vi "10-Tap 8-Bit Camera with DRAM(Host).vi"() -> ()   [LabVIEW 2014]
doc: "This is the host VI for the 10-Tap 8-Bit Camera with DRAM example. This example demonstrates how to acquire images from a 10-tap, 8-bit, extended configuration, Camera Link camera and display the images on the host. This example supports area scan and line scan cameras for both continuous and finite acquisitions.\n\nThis example also demonstrates the use of DRAM as a frame buffer for very high speed acquisitions. Data packing and flow-control are also employed to maximize use of the available DRAM and FIFOs in terms of both memory space and performance.\n\nAdditionally, the example demonstrates the serial server, which allows third-party camera configuration utilities to communicate with the camera using the Camera Link serial interface while this VI is running."
uses:
  <vilib>/userdefined/High Color/nirio_resource_hc.ctl
  <vilib>/FPGAPlugInAG/PCIe-1473R/niLvFpga_Open_PCIe-1473R.vi
  <vilib>/rvi/interface/common/dynamic/niFpgaDynamicAddResources.vi
  <vilib>/FPGAPlugInAG/Dynamic/niLvFpga_Reset_Dynamic.vi
  <vilib>/Utility/error.llb/Error Cluster From Error Code.vi
  <vilib>/rvi/errors/niLvFpgaAdjustHostInterfaceError.vi
  <vilib>/FPGAPlugInAG/Dynamic/niLvFpga_Run_Dynamic.vi
  <vilib>/rvi/interface/common/niFpgaWaitOnOcc.vi
  <vilib>/DAQmx/write.llb/DAQmx Write (Analog DBL 1Chan 1Samp).vi
  <vilib>/FPGAPlugInAG/Dynamic/niLvFpga_Close_Dynamic.vi
  <vilib>/rvi/interface/nirviOpenFPGA/nirviOpenFPGA.xnode
  FPGA Bitfiles/10-Tap8-bitCamer_FPGATarget_10-Tap8-bitCamer_C490DC32.lvbitx
  10-Tap 8-Bit Camera with DRAM(FPGA).vi
  <vilib>/rvi/interface/nirviMethod/nirviMethod.xnode
  <vilib>/rvi/interface/nirviReadWriteControl/nirviReadWriteControl.xnode
  <vilib>/rvi/interface/nirviCloseFPGA/nirviCloseFPGA.xnode
  <vilib>/rvi/interface/Simulation/niFpgaSimulationCallBeginRW.vi
  <vilib>/rvi/errors/niLvFpgaMergeErrorWithErrorCode.vi
  NiFpgaLv.dll
  <vilib>/FPGAPlugInAG/Dynamic/niLvFpga_ReadFifo_Dynamic.vi
  <vilib>/FPGAPlugInAG/Dynamic/niLvFpga_ConfigureFifo_Dynamic.vi
  <vilib>/FPGAPlugInAG/Dynamic/niLvFpga_StartFifo_Dynamic.vi
panel:
  out "测得角度":dbl
  out "?":dbl
  out "目标中心":dbl
  out "?":dbl
  out "边框中心":dbl
  in  "BodyLength":dbl=10.0
  in  "FishLength":u16=300
  out "?":u16
  out "?":u16
  out "Xmax":u16
  out "边框":u16
  in  "Y":dbl=384.0 format="%#_13g"
  in  "X":dbl=520.0 format="%#_13g"
  in  "offset":dbl=150.0
  in  "SpeedFactor":dbl=1.0
  out "数量":i32
  out "?":fxp<+,32,16> format="%.21g"
  out "测得中心":fxp<+,32,16> format="%.21g"
  in  "Threshold":u8=96
  in  "DMA Buffer Size\n(In Images)":u32=64 caption="DMA Buffer Size"
  in  "Signal Mapping":T1(ring)=enum."Basler 10-tap"
  out "Acq In Progress":bool
  in  "Line Scan":bool
  in  "Frames To Acquire":u32 caption="Frames To Acquire\n(0 = infinite)"
  in  "Cancel":bool
  out "Acq'd Frame Width":u32
  in  "Stopped":bool
  in  "RIO Device":T2="Horizontal"
  out "DMA Write Timeout":bool
  in  "Start Serial Server":bool=TRUE
  out "Frames Acq'd":u32
  out "Acq'd Frame Height":u32
  out "Image":T3(plugin-control)
  in  "Acquire":bool
  in  "Stop":bool
  in  "Image Height":u32=768 max=65535
  in  "Image Width":u32=1040 max=65535 step=40
  out "Initialized":bool
  # "这个值越小，那么即便是比较小的距离也会移动较快，参考值50"
  # "与速度有关的乘方因子，必须是奇数，参考值1"
  # "目标位置"
  # "期望中心位置"
  # "鱼的身体长度，如果边界大小超过这个值，就放弃此次补偿计算，参考值800"
  # "希望补偿的长度，一般应小于鱼的身体长度，参考值10"
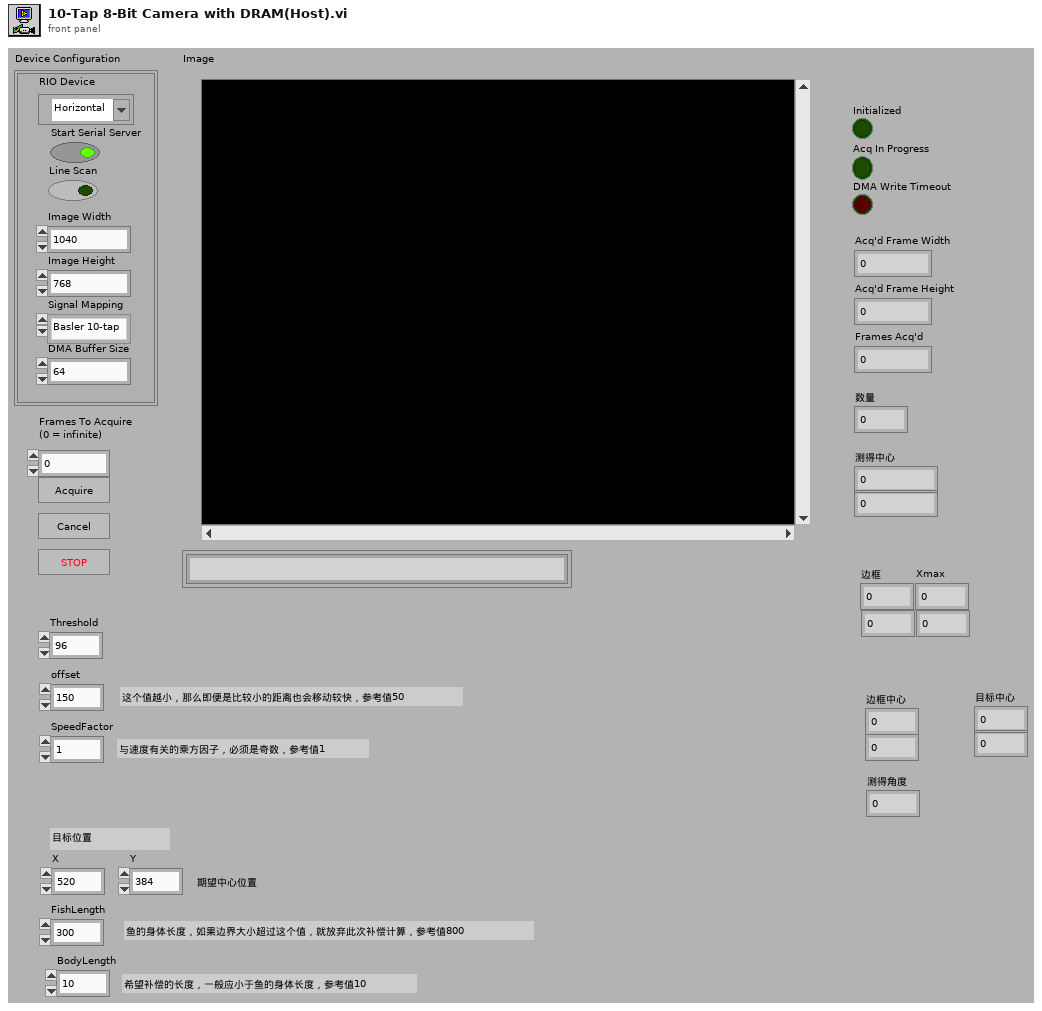
[diagram p1: front panel]
types:
  T1 = enum8{"Standard", "Basler 10-tap", "Vosskühler 10-tap"}
  T2 = typedef "nirio_resource_hc.ctl" = tag
  T3 = typedef "IMAQ Image.ctl" = refnum<image>
  T4 = typedef "Image Type" = u32
  T5 = enum16{"big-endian, network order", "native, host order", "little-endian"}
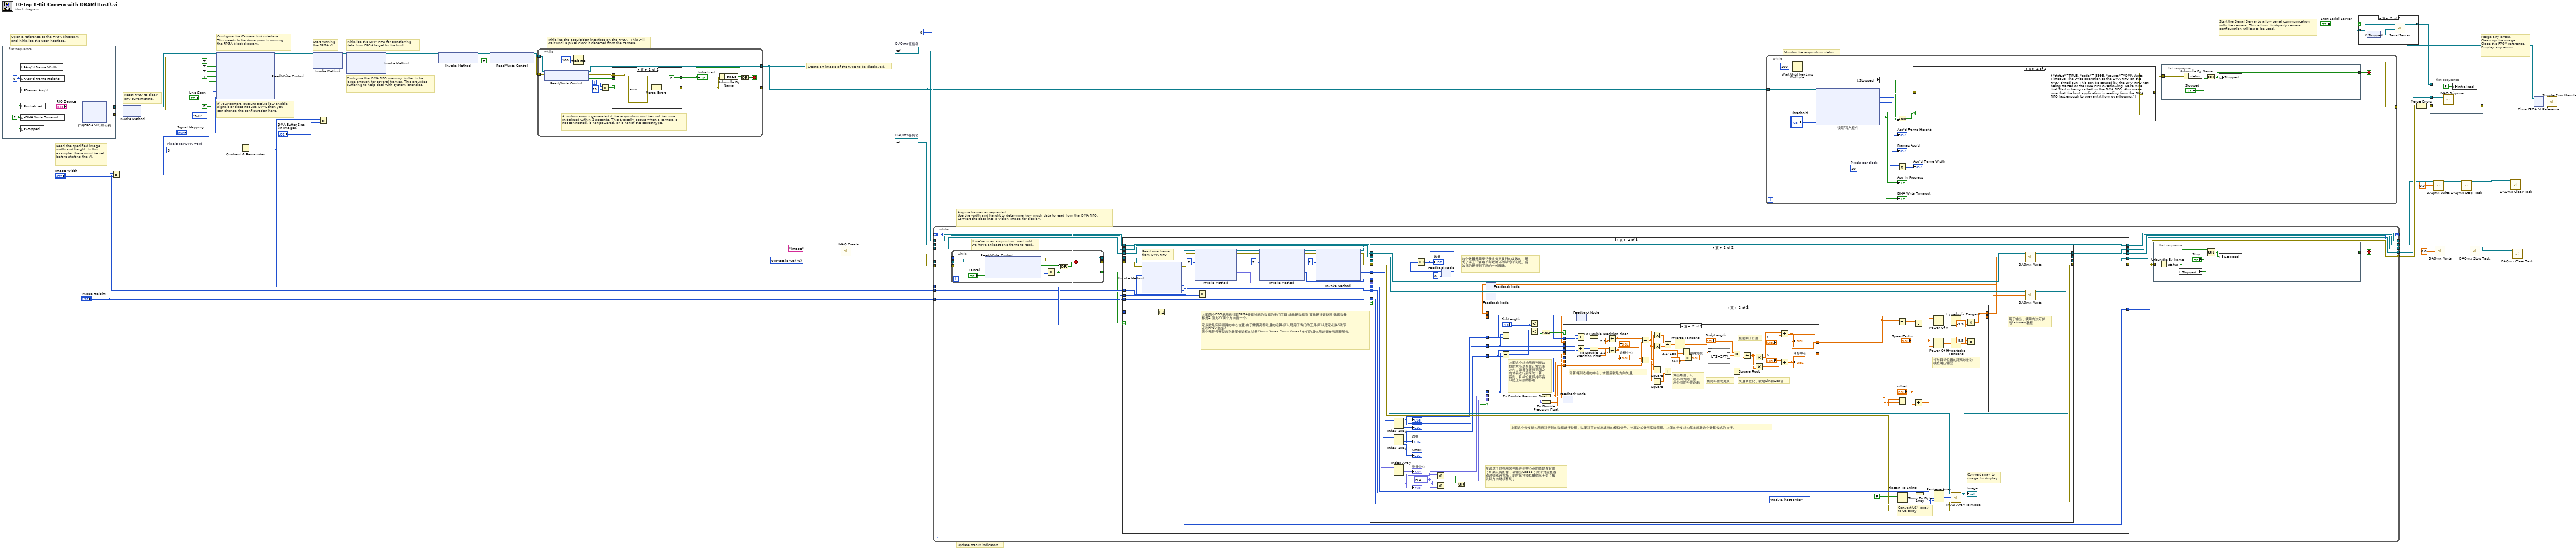
[diagram p0: block diagram]
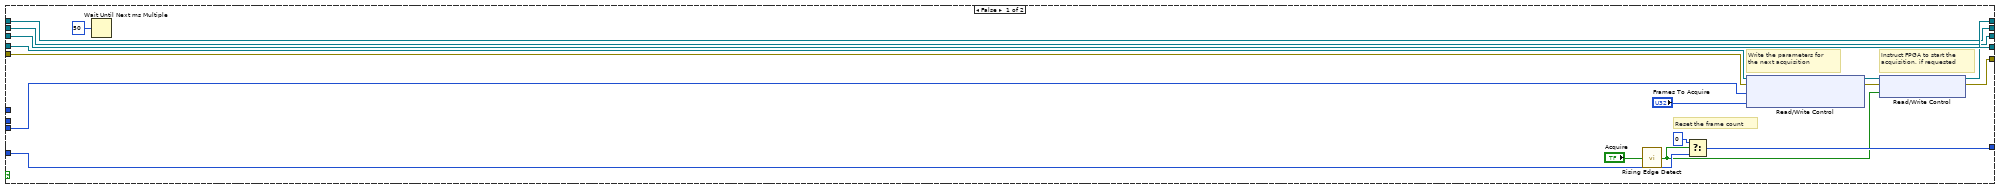
[diagram p4: hidden frame]
diagram:
  w9 = refnum<k21> "Stage_Y"  # DAQmx任务名
  w10 = refnum<k21> "Stage_X"  # DAQmx任务名
  w15 = u32 8  # Pixels per DMA word
  w52 = T4 0 items=["Grayscale (U8)", "Grayscale (I16)", "Grayscale (SGL)", "Complex (CSG)", "RGB (U32)", "HSL (U32)", "RGB (U64)", "Grayscale (U16)"] ("Image Type")
  # "Update status indicators"
  # "If your camera outputs active-low enable\nsignals or does not use DVAL then you \ncan change the configuration here."
  # "Configure the DMA FIFO memory buffer to be\nlarge enough for several frames. This provides\nbuffering to help deal with system latencies."
  # "Start running\nthe FPGA VI."
  # "Reset FPGA to clear\nany current state."
  # "Read the specified image\nwidth and height. In this\nexample, these must be set\nbefore starting the VI."
  # "Merge any errors.\nClean up the image.\nClose the FPGA reference.\nDisplay any errors."
  # "Acquire frames as requested.\nUse the width and height to determine how much data to read from the DMA FIFO.\nConvert the data into a Vision Image for display."
  # "Monitor the acquisition status"
  # "Start the Serial Server to allow serial communication\nwith the camera. This allows third-party camera\nconfiguration utilites to be used."
  # "Create an image of the type to be displayed."
  # "Initialize the acquisition interface on the FPGA.  This will\nwait until a pixel clock is detected from the camera."
  # "Initialize the DMA FIFO for transferring\ndata from FPGA target to the host."
  # "Configure the Camera Link interface.\nThis needs to be done prior to running\nthe FPGA block diagram."
  # "Open a reference to the FPGA bitstream\nand initialize the user interface."
  n1 = flat-sequence {
    tunnel: [w58] -> w43
    tunnel: [w57] -> w56
    frame #0 {
      w61 = u32 0 ("Num Lines Acq'd")
      w60 = FALSE ("stop")
      n2 = local write "Acq'd Frame Width"(w61) -> ()
      n3 = local write "Acq'd Frame Height"(w61) -> ()
      n4 = local write "Frames Acq'd"(w61) -> ()
      n5 = local write "Initialized"(w60) -> ()
      n6 = local write "DMA Write Timeout"(w60) -> ()
      n7 = local write "Stopped"(w60) -> ()
      n8 = xnode "打开FPGA VI引用句柄"("资源名称"="RIO Device") -> ("FPGA VI引用输出"=w58:refnum<k20>, "错误输出"=w57:errorcluster)  [unwired: 1 in]
    }
  }
  n9 = Multiply(x="Image Height", y="Image Width") -> (x*y=w14:u32)
  n10 = xnode "Invoke Method"("FPGA VI引用输入"=w43, "错误输入"=w56) -> ("FPGA VI引用输出"=w32:refnum<k20>, "错误输出"=w35:errorcluster)
  n11 = xnode "Read/Write Control"("FPGA VI引用输入"=w32, "错误输入"=w35, "CL Config.FVAL Active High"=TRUE ("IO Module Config.CL FVAL Active High"), "CL Config.LVAL Active High"=TRUE ("IO Module Config.CL LVAL Active High"), "CL Config.DVAL Active High"=TRUE ("IO Module Config.CL DVAL Active High"), "CL Config.Spare Active High"=TRUE ("IO Module Config.CL Spare Active High"), "CL Config.Line Scan"="Line Scan", "Acq Control.Ignore DVAL"=FALSE ("CL Config.Line Scan"), "CL Config.Configuration"=enum8{"Base", "Medium", "Full"}."Full", "CL Config.Signal Mapping"="Signal Mapping") -> ("FPGA VI引用输出"=w36:refnum<k20>, "错误输出"=w34:errorcluster)
  n12 = Quotient & Remainder(x=w14, y=w15) -> (floor(x/y)=w13:u32)  [unwired: 1 out]
  n13 = xnode "Invoke Method"("FPGA VI引用输入"=w36, "错误输入"=w34) -> ("FPGA VI引用输出"=w12:refnum<k20>, "错误输出"=w11:errorcluster)  [unwired: 1 in]
  n14 = Multiply(x=w13, y="DMA Buffer Size\n(In Images)") -> (x*y=w26:u32)
  n15 = xnode "Invoke Method"("FPGA VI引用输入"=w12, "错误输入"=w11, "请求的深度"=w26) -> ("FPGA VI引用输出"=w42:refnum<k20>, "错误输出"=w41:errorcluster)  [unwired: 1 out]
  n16 = xnode "Invoke Method"("FPGA VI引用输入"=w42, "错误输入"=w41) -> ("FPGA VI引用输出"=w27:refnum<k20>, "错误输出"=w40:errorcluster)
  n17 = xnode "Read/Write Control"("FPGA VI引用输入"=w27, "错误输入"=w40, "Acq Control.Initialize"=TRUE ("Arm Acquisition")) -> ("FPGA VI引用输出"=w55:refnum<k20>, "错误输出"=w54:errorcluster)
  n18 = while {
    tunnel: w55 -> [w69]
    tunnel: w54 -> [w68]
    tunnel: [w67] -> w23
    tunnel: [w71] -> w22
    i -> [w63]
    stop <- w74 stop-if-true
    # "A custom error is generated if the acquisition unit has not become\ninitialized within 2 seconds. This typically occurs when a camera is\nnot connected, is not powered, or is not of the correct type."
    n19 = xnode "Read/Write Control"("FPGA VI引用输入"=w69, "错误输入"=w68) -> ("FPGA VI引用输出"=w67:refnum<k20>, "错误输出"=w66:errorcluster, "Acq Status.Initialized"=w65:bool)
    n20 = Wait (ms)(milliseconds to wait=u32 100) -> ()  [unwired: 1 out]
    n21 = Greater?(x=w63, y=20) -> (0:w64:bool)
    n22 = case shown="真" w64 {
      tunnel: [w76 FALSE] -> w70
      tunnel: w65 -> [w76 _]
      tunnel: w66 -> [w75 w78]
      tunnel: [w75 w80] -> w71
      frame False {
      }
      frame True {
        n23 = Merge Errors(w78, errorcluster {"status"=TRUE, "code"=-8999, "source"="Acquisition Initialization: This error typically occurs when a camera is not properly connected, is not powered, or is not of the correct type."} ("error in")) -> (w80:errorcluster)
      }
    }
    "Initialized" <- w70
    n24 = Unbundle By Name(w71) -> ("status"=w73:bool)
    n25 = Or(x=w73, y=w70) -> (x .or. y?=w74:bool)
  }
  n26 = call "IMAQ Create"("Image Name"="Image", "Image Type"=w52, "error in (no error)"=w22) -> ("New Image"=w19:T3, "error out"=w18:errorcluster)  [unwired: 2 in]
  n27 = while {
    tunnel: w23 -> [w91]
    tunnel: w18 -> [w90]
    tunnel: w13 -> [w99]
    tunnel: "Image Height" -> [w98]
    tunnel: "Image Width" -> [w97]
    tunnel: w19 -> [w96]
    tunnel: [w94] -> w38
    tunnel: [w95] -> w51
    tunnel: [w92] -> w46
    shift-right: [w86] -> _
    shift-left: u32 0 -> [w85]
    tunnel: w10 -> [w84]
    tunnel: w9 -> [w83]
    tunnel: [w82] -> w8
    tunnel: [w81] -> w6
    stop <- w93 stop-if-true
    # "If we're in an acquisition, wait until\nwe have at least one frame to read."
    n28 = while {
      tunnel: w91 -> [w106]
      tunnel: w90 -> [w105]
      tunnel: [w103] -> w89
      tunnel: [w104] -> w88
      tunnel: w85 -> [w109]
      tunnel: [w107] -> w87
      stop <- w108 stop-if-true
      n29 = xnode "Read/Write Control"("FPGA VI引用输入"=w106, "错误输入"=w105, "Acq Control.Cancel Acq"="Cancel") -> ("FPGA VI引用输出"=w104:refnum<k20>, "错误输出"=w103:errorcluster, "Acq Status.Acq In Progress"=w102:bool, "Acq Status.Frames Acq'd"=w101:u32)
      n30 = Greater?(x=w101, y=w109) -> (0:w107:bool)
      n31 = Compound Arithmetic op=OR(invert w102, w107) -> (w108:bool)
    }
    n32 = case shown="真" w87 {
      tunnel: w88 -> [w127 w157]
      tunnel: w89 -> [w126 w156]
      tunnel: w99 -> [_ w150]
      tunnel: w98 -> [w120 w162]
      tunnel: w97 -> [_ w161]
      tunnel: w96 -> [w131 w160]
      tunnel: [w122 w159] -> w94
      tunnel: [w125 w136] -> w95
      tunnel: [w131 w158] -> w92
      tunnel: w85 -> [w128 w155]
      tunnel: [w130 w154] -> w86
      tunnel: w84 -> [w116 w145]
      tunnel: w83 -> [w115 w144]
      tunnel: [w116 w143] -> w82
      tunnel: [w115 w142] -> w81
      frame False {
        # "Reset the frame count"
        # "Instruct FPGA to start the\nacquisition, if requested"
        # "Write the parameters for\nthe next acquisition"
        n33 = Wait Until Next ms Multiple(millisecond multiple=u32 50) -> ()  [unwired: 1 out]
        n34 = call "Rising Edge Detect.vi"("Input"="Acquire") -> ("Pulse"=w117:bool)  [unwired: 4 in]
        n35 = Select(t=u32 0, s=w117, f=w128) -> (s? t:f=w130:u32)
        n36 = xnode "Read/Write Control"("FPGA VI引用输入"=w127, "错误输入"=w126, "Acq Control.Line Scan Height"=w120, "Acq Control.Frames To Acq"="Frames To Acquire") -> ("FPGA VI引用输出"=w124:refnum<k20>, "错误输出"=w123:errorcluster)
        n37 = xnode "Read/Write Control"("FPGA VI引用输入"=w124, "错误输入"=w123, "Acq Control.Acquire"=w117) -> ("FPGA VI引用输出"=w125:refnum<k20>, "错误输出"=w122:errorcluster)
      }
      frame True {
        # "上面四个FIFO是用来读取FPGA传输过来的数据的专门工具,绿线是数据流,黄线是错误处理.元素数量\n都是2 因为XY两个方向各一个.\n\n定点数是实际测得的中心位置,由于需要高吞吐量的运算,所以是用了专门的工具,所以是定点数.(该节\n点在FPGA里面.)\n两个无符号整型分别是图像边框的边界(Xmin,Xmax,Ymin,Ymax),他们的具体用途请参考原理部分。"
        # "Read one frame\nfrom DMA FIFO"
        n38 = xnode "Invoke Method"("FPGA VI引用输入"=w157, "错误输入"=w156, "元素数量"=w150) -> ("FPGA VI引用输出"=w149:refnum<k20>, "错误输出"=w148:errorcluster, "数据"=w153:u64[], "剩余元素"=w151:u32)  [unwired: 1 in]
        n39 = Increment(x=w155) -> (x+1=w154:u32)
        n40 = xnode "Invoke Method"("FPGA VI引用输入"=w149, "错误输入"=w148, "元素数量"=u32 2) -> ("FPGA VI引用输出"=w138:refnum<k20>, "错误输出"=w141:errorcluster, "数据"=w146:fxp<+,32,16>[])  [unwired: 1 in, 1 out]
        n41 = Less?(x=w151, y=w150) -> (x < y?=w152:bool)
        n42 = xnode "Invoke Method"("FPGA VI引用输入"=w138, "错误输入"=w141, "元素数量"=u32 2) -> ("FPGA VI引用输出"=w137:refnum<k20>, "错误输出"=w140:errorcluster, "数据"=w133:u16[])  [unwired: 1 in, 1 out]
        n43 = xnode "Invoke Method"("FPGA VI引用输入"=w137, "错误输入"=w140, "元素数量"=u32 2) -> ("FPGA VI引用输出"=w136:refnum<k20>, "错误输出"=w139:errorcluster, "数据"=w132:u16[])  [unwired: 1 in, 1 out]
        n44 = case shown="真" w152 {
          tunnel: w162 -> [_ w202]
          tunnel: w161 -> [_ w201]
          tunnel: w160 -> [w166 w200]
          tunnel: w139 -> [w165 w199]
          tunnel: [w165 w191] -> w159
          tunnel: [w166 w198] -> w158
          tunnel: w153 -> [_ w195]
          tunnel: w146 -> [_ w190]
          tunnel: w145 -> [w164 w189]
          tunnel: w144 -> [w163 w188]
          tunnel: [w164 w187] -> w143
          tunnel: [w163 w186] -> w142
          tunnel: w133 -> [_ w172]
          tunnel: w132 -> [_ w171]
          frame False {
            # "Do not display the image if we're falling behind in the acquisition."
          }
          frame True {
            w185 = fxp<+,32,16> 10000.0 ("y")
            # "用于输出，使用方法可参\n考Labview教程"
            # "左边这个结构用来判断得到中心点的值是否合理\n（如果没有图像，会输出65533）此时对应鱼游\n动过快离开视场，此时保持模拟量输出不变（按\n失踪方向继续移动）"
            # "上面这个分支结构用来对得到的数据进行处理，以便对平台输出适当的模拟信号。计算公式参考实验原理。上面的分支结构基本就是这个计算公式的执行。"
            # "这个数量是用来记录此分支执行的次数的，是\n为了手工计算每个有效循环的平均时间的。有\n效指的是得到了新的一帧图像。"
            # "Convert U64 array\nto U8 array"
            # "Convert array to\nimage for display"
            n45 = Index Array(array=w171) -> (element #1=w167:u16, element #2=w168:u16)  [unwired: 2 in]
            "?" <- w167
            "?" <- w168
            n46 = Index Array(array=w172) -> (element #1=w169:u16, element #2=w170:u16)  [unwired: 2 in]
            "边框" <- w169
            "Xmax" <- w170
            n47 = Index Array(array=w190) -> (element #1=w181:fxp<+,32,16>, element #2=w180:fxp<+,32,16>)  [unwired: 2 in]
            "测得中心" <- w181
            "?" <- w180
            n48 = Less?(x=w181, y=w185) -> (x < y?=w183:bool)
            n49 = Less?(x=w180, y=w185) -> (x < y?=w184:bool)
            n50 = feedback #1(0) -> (w174:i32)
            n51 = Increment(x=w174) -> (x+1=w173:i32)
            "数量" <- w173
            n52 = feedback-in #1(w173) -> ()
            n53 = Or(x=w183, y=w184) -> (x .or. y?=w182:bool)
            n54 = feedback #2() -> (w177:dbl)  [unwired: 1 in]
            n55 = feedback #3() -> (w176:dbl)  [unwired: 1 in]
            n56 = case shown="真" w182 {
              tunnel: w181 -> [_ w236]
              tunnel: w180 -> [_ w235]
              tunnel: [w204 w234] -> w179
              tunnel: [w203 w233] -> w178
              tunnel: w177 -> [w204 _]
              tunnel: w176 -> [w203 _]
              tunnel: w170 -> [_ w216]
              tunnel: w169 -> [_ w215]
              tunnel: w168 -> [_ w214]
              tunnel: w167 -> [_ w213]
              frame False {
              }
              frame True {
                # "将与目标位置的距离映射为\n模拟电压输出"
                # "上面这个结构用来判断边\n框的大小是否在正常范围\n之内，如果在正常范围之\n内才会进行后来的计算，\n否则，目标位置保持不变\n以防止杂质的影响"
                n57 = Subtract(x=w214, y=w213) -> (x-y=w217:u16)
                n58 = Subtract(x=w216, y=w215) -> (x-y=w218:u16)
                n59 = Less?(x=w217, y="FishLength") -> (x < y?=w219:bool)
                n60 = Less?(x=w218, y="FishLength") -> (x < y?=w220:bool)
                n61 = And(x=w220, y=w219) -> (x .and. y?=w221:bool)
                n62 = To Double Precision Float(number=w236) -> (double precision float=w212:dbl)
                n63 = To Double Precision Float(number=w235) -> (double precision float=w211:dbl)
                n64 = feedback #4() -> (w207:dbl)  [unwired: 1 in]
                n65 = feedback #5() -> (w209:dbl)  [unwired: 1 in]
                n66 = case shown="真" w221 {
                  tunnel: w216 -> [_ w274]
                  tunnel: w215 -> [_ w273]
                  tunnel: w214 -> [_ w271]
                  tunnel: w213 -> [_ w270]
                  tunnel: w212 -> [_ w267]
                  tunnel: w211 -> [_ w265]
                  tunnel: [w238 w259] -> w210
                  tunnel: [w237 w258] -> w208
                  tunnel: w209 -> [w238 _]
                  tunnel: w207 -> [w237 _]
                  frame False {
                  }
                  frame True {
                    # "横向补偿的更长"
                    # "提前乘了长度"
                    # "矢量单位化，就是Sin和Cos值"
                    # "算出角度，以\n在不同方向上使\n用不同的补偿距离"
                    # "计算得到边框的中心，求差后就是方向矢量。"
                    n67 = Add(x=w271, y=w270) -> (x+y=w272:u16)
                    n68 = Add(x=w274, y=w273) -> (x+y=w275:u16)
                    n69 = To Double Precision Float(number=w272) -> (double precision float=w252:dbl)
                    n70 = To Double Precision Float(number=w275) -> (double precision float=w253:dbl)
                    n71 = Divide(x=w252, y=2.0) -> (x/y=w266:dbl)
                    "?" <- w266
                    n72 = Divide(x=w253, y=2.0) -> (x/y=w268:dbl)
                    "边框中心" <- w268
                    n73 = Subtract(x=w266, y=w265) -> (x-y=w247:dbl)
                    n74 = Subtract(x=w268, y=w267) -> (x-y=w249:dbl)
                    n75 = Square(x=w249) -> (x^2=w264:dbl)
                    n76 = Square(x=w247) -> (x^2=w263:dbl)
                    n77 = Absolute Value(x=w249) -> (abs(x)=w250:dbl)
                    n78 = Absolute Value(x=w247) -> (abs(x)=w248:dbl)
                    n79 = Divide(x=w250, y=w248) -> (x/y=w251:dbl)
                    n80 = Add(x=w264, y=w263) -> (x+y=w262:dbl)
                    n81 = Inverse Tangent(1:w251) -> (0:w244:dbl)
                    n82 = Divide(x=w244, y=3.14159) -> (x/y=w242:dbl)
                    n83 = Multiply(x=w242, y=360.0) -> (x*y=→"测得角度":dbl)
                    n84 = formula code="L=3+2*T;"("T"=w244) -> ("L"=w243:dbl)
                    n85 = Multiply(x="BodyLength", y=w243) -> (x*y=w245:dbl)
                    n86 = Square Root(x=w262) -> (sqrt(x)=w254:dbl)
                    n87 = Divide(x=w245, y=w254) -> (x/y=w246:dbl)
                    n88 = Multiply(x=w246, y=w247) -> (x*y=w255:dbl)
                    n89 = Multiply(x=w249, y=w246) -> (x*y=w256:dbl)
                    n90 = Add(x=w255, y="Y") -> (x+y=w258:dbl)
                    "?" <- w258
                    n91 = Add(x="X", y=w256) -> (x+y=w259:dbl)
                    "目标中心" <- w259
                  }
                }
                n92 = feedback-in #4(w208) -> ()
                n93 = feedback-in #5(w210) -> ()
                n94 = Subtract(x=w210, y=w212) -> (x-y=w232:dbl)
                n95 = Subtract(x=w211, y=w208) -> (x-y=w231:dbl)
                n96 = Divide(x=w232, y="offset") -> (x/y=w226:dbl)
                n97 = Divide(x=w231, y="offset") -> (x/y=w224:dbl)
                n98 = Power Of X(1:w226, 2:"SpeedFactor") -> (0:w227:dbl)
                n99 = Power Of X(1:w224, 2:"SpeedFactor") -> (0:w225:dbl)
                n100 = Hyperbolic Tangent(1:w227) -> (0:w230:dbl)
                n101 = Hyperbolic Tangent(1:w225) -> (0:w229:dbl)
                n102 = Multiply(x=w230, y=-9.5) -> (x*y=w234:dbl)
                n103 = Multiply(x=-9.5, y=w229) -> (x*y=w233:dbl)
              }
            }
            n104 = feedback-in #2(w179) -> ()
            n105 = feedback-in #3(w178) -> ()
            n106 = Flatten To String(anything=w195, prepend array or string size? (T)=FALSE, byte order (0:big-endian, network order)=T5."native, host order") -> (data string=w193:string)  [unwired: 1 in, 2 out]
            n107 = String To Byte Array(string=w193) -> (unsigned byte array=w192:u8[])
            n108 = Reshape Array(w192, w202, w201) -> (w197:u8[][])
            n109 = call "IMAQ ArrayToImage"("error in (no error)"=w199, "Image Pixels (U8)"=w197, "Image"=w200) -> ("error out"=w191:errorcluster, "Image Out"=w198:T3)  [unwired: 7 in]
            "Image" <- w198
            n110 = call-poly <vilib>:"DAQmx Write.vi"("task/channels in"=w189, "data"=w179) -> ("task out"=w187:refnum<k21>)  [unwired: 11 in, 2 out]
            n111 = call-poly <vilib>:"DAQmx Write.vi"("task/channels in"=w188, "data"=w178) -> ("task out"=w186:refnum<k21>)  [unwired: 11 in, 2 out]
          }
        }
      }
    }
    n112 = flat-sequence {
      tunnel: w94 -> [w112]
      tunnel: [w111] -> w93
      frame #0 {
        n113 = Unbundle By Name(w112) -> ("status"=w113:bool)
        n114 = local read "Stopped"() -> (w110:bool)
        n115 = Compound Arithmetic op=OR(w113, "Stop", w110) -> (w111:bool)
        n116 = local write "Stopped"(w111) -> ()
      }
    }
  }
  n117 = while {
    tunnel: w23 -> [w288]
    tunnel: [w291] -> w37
    stop <- w290 stop-if-true
    w281 = u32 10  # Pixels per clock
    n118 = Wait Until Next ms Multiple(millisecond multiple=u32 100) -> ()  [unwired: 1 out]
    n119 = xnode "读取/写入控件"("FPGA VI引用输入"=w288, "Threshold"="Threshold") -> ("错误输出"=w287:errorcluster, "Acq Status.Lines Per Frame"=→"Acq'd Frame Height":u32, "Acq Status.Frames Acq'd"=→"Frames Acq'd":u32, "Acq Status.Clocks Per Line"=w282:u32, "Acq Status.Acq In Progress"=→"Acq In Progress":bool, "Acq Status.DMA Write Timeout"=w279:bool)  [unwired: 1 in, 1 out]
    "DMA Write Timeout" <- w279
    n120 = local read "Stopped"() -> (w278:bool)
    n121 = Multiply(x=w282, y=w281) -> (x*y=→"Acq'd Frame Width":u32)
    n122 = Compound Arithmetic op=AND(w279, invert w278) -> (w280:bool)
    n123 = case shown="真" w280 {
      tunnel: w287 -> [w296 _]
      tunnel: [w296 errorcluster {"status"=TRUE, "code"=-8999, "source"="DMA Write Timeout: The write operation to the DMA FIFO on the FPGA timed out. This can be caused by the DMA FIFO not being started or the DMA FIFO overflowing. Make sure that Start is being called on the DMA FIFO. Also make sure that the host application is reading from the DMA FIFO fast enough to prevent it from overflowing."} ("error out")] -> w291
      frame False {
      }
      frame True {
      }
    }
    n124 = flat-sequence {
      tunnel: w291 -> [w295]
      tunnel: [w293] -> w290
      frame #0 {
        n125 = Unbundle By Name(w295) -> ("status"=w294:bool)
        n126 = Or(x=w294, y="Stopped") -> (x .or. y?=w293:bool)
        n127 = local write "Stopped"(w293) -> ()
      }
    }
  }
  n128 = case shown="真" "Start Serial Server" {
    tunnel: [_ w298] -> w44
    tunnel: w23 -> [_ w299]
    frame False {
    }
    frame True {
      n129 = control-ref of="Stopped"() -> (w300:refnum<vi>)
      n130 = call "SerialServer.vi"("Stop Refnum"=w300, "FPGA VI Reference In"=w299) -> ("FPGA VI Reference Out"=w298:refnum<k20>)  [unwired: 5 in]
    }
  }
  n131 = Merge Errors(w38, w37) -> (w39:errorcluster)
  n132 = flat-sequence {
    tunnel: w39 -> [w302]
    tunnel: [w302] -> w48
    tunnel: w46 -> [w303]
    tunnel: w44 -> [_]
    frame #0 {
      n133 = call "IMAQ Dispose"("Image"=w303) -> ()  [unwired: 5 in, 1 out]
      n134 = local write "Initialized"(FALSE ("Module Enabled")) -> ()
    }
  }
  n135 = call-poly <vilib>:"DAQmx Write.vi"("task/channels in"=w8, "data"=0.0) -> ("task out"=w4:refnum<k21>)  [unwired: 11 in, 2 out]
  n136 = call-poly <vilib>:"DAQmx Write.vi"("task/channels in"=w6, "data"=0.0) -> ("task out"=w2:refnum<k21>)  [unwired: 11 in, 2 out]
  n137 = call <vilib>:"DAQmx Stop Task.vi"("task/channels in"=w4) -> ("task out"=w7:refnum<k21>)  [unwired: 13 in, 1 out]
  n138 = call <vilib>:"DAQmx Stop Task.vi"("task/channels in"=w2) -> ("task out"=w5:refnum<k21>)  [unwired: 13 in, 1 out]
  n139 = call <vilib>:"DAQmx Clear Task.vi"("task in"=w7) -> ()  [unwired: 14 in, 1 out]
  n140 = call <vilib>:"DAQmx Clear Task.vi"("task in"=w5) -> ()  [unwired: 14 in, 1 out]
  n141 = xnode "Close FPGA VI Reference"("FPGA VI引用输入"=w51, "错误输入"=w48) -> ("错误输出"=w45:errorcluster)
  n142 = call <vilib>:"Simple Error Handler.vi"("error in (no error)"=w45) -> ()  [unwired: 4 in, 5 out]
